vi "Build Schedule.vi"(10 "Number of Test Cases":i32, 11 "Number of Test Runners":i32) -> (3 "Schedule":i32[](array[numeric]))   [LabVIEW 2020, in "Test Runner.lvclass"]
uses:
  Test Runner.lvclass
  Test Runner.lvclass/Test Runner.ctl
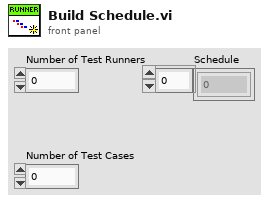
[diagram p1: front panel]
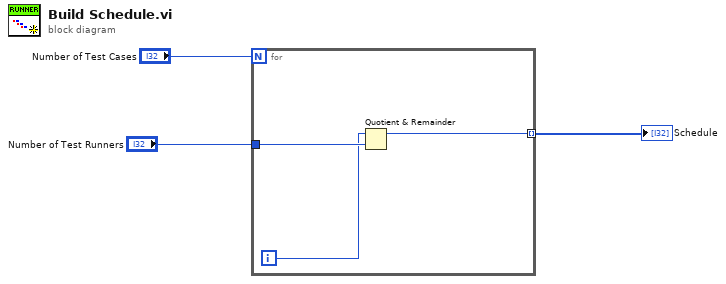
[diagram p0: block diagram]
diagram:
  n1 = for {
    N: "Number of Test Cases" -> [_]
    tunnel: "Number of Test Runners" -> [w6]
    tunnel: [w4] -> w1 mode=indexing
    i -> [w5]
    n2 = Quotient & Remainder(x=w5, y=w6) -> (x-y*floor(x/y)=w4:i32)  [unwired: 1 out]
  }
  "Schedule" <- w1
